vi "setUp.vi"(8 "error in (no error)":errorcluster, 11 "reference in":refnum<class "Test Status Updater.lvclass">) -> (0 "error out":errorcluster, 3 "reference out":refnum<class "Test Status Updater.lvclass">)   [LabVIEW 2014, in "Test Status Updater.lvclass"]
doc: "setUp runs prior to the test method during test execution. Use this method to initialize any object data required by your tests."
uses:
  Test Status Updater.lvclass
  Test Status Updater.lvclass/Test Status Updater.ctl
  <vilib>/addons/_JKI Toolkits/VI Tester/TestCase.llb/TestCase.lvclass
  Core/Shared/Classes/Status Updater/Status Updater.lvclass
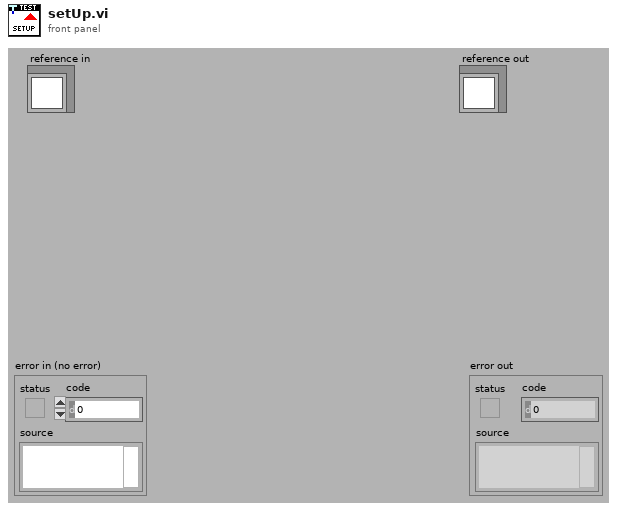
[diagram p1: front panel]
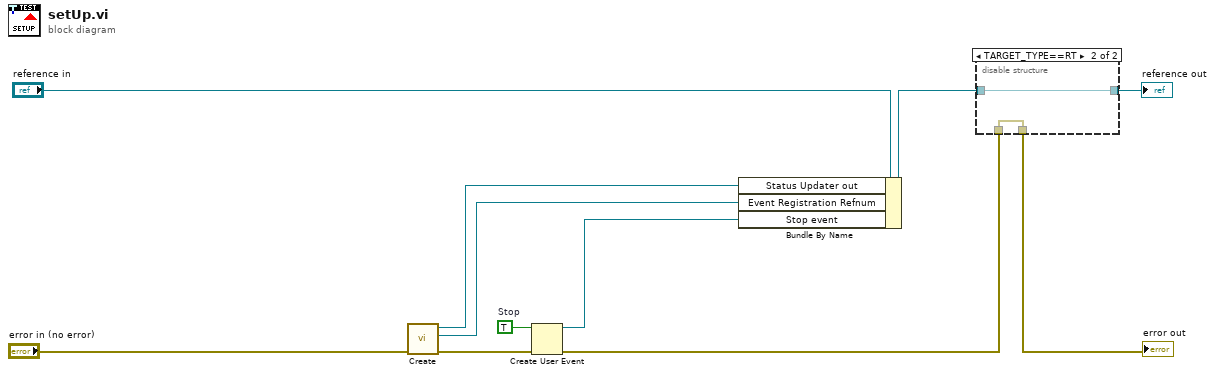
[diagram p0: block diagram]
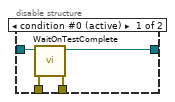
[diagram p2: hidden frame]
diagram:
  w4 = TRUE  # Stop
  n1 = call "Create.vi"("error in (no error)"="error in (no error)") -> ("error out"=w3:errorcluster, "Event Registration Refnum"=w5:refnum<event-registration>, "Status Updater out"=w6:refnum<class "Status Updater.lvclass">)  [unwired: 8 in]
  n2 = Create User Event(user event datatype=w4, error in=w3) -> (user event=w1:refnum<user-event>, error out=w2:errorcluster)
  n3 = Bundle By Name(cluster="reference in", "Status Updater out"=w6, "Event Registration Refnum"=w5, "Stop event"=w1) -> (w8:refnum<class "Test Status Updater.lvclass">)
  n4 = disable-structure shown="TARGET_TYPE==RT" {
    disable-tunnel: w2 -> [w15 w16]
    disable-tunnel: [w14 w16] -> w11
    disable-tunnel: [w13 w17] -> w9
    disable-tunnel: w8 -> [w12 w17]
    frame condition #0 (active) {
      n5 = call <vilib>:"WaitOnTestComplete.vi"("error in (no error)"=w15, "TestCase in"=w12) -> ("error out"=w14:errorcluster, "TestCase out"=w13:refnum<class "Test Status Updater.lvclass">)  [unwired: 8 in]
    }
    frame condition #1 {
    }
  }
  "error out" <- w11
  "reference out" <- w9
